vi "PicoScope2000ExampleAWG.vi"() -> ()   [LabVIEW 2010]
panel:
  in  "Waveform Settings":T1={"Arbirary waveform file path"=path "", "Sweep Type"=0, "Sweeps"=0, "Wave Type"=0, "Start Frequency"=1000.0, "Stop Frequency"=1000.0, "Increment (Hz)"=0.0, "Dwell Time (seconds)"=0.0, "Offset Voltage (uV)"=0, "Peak to Peak (uV)"=2000000} {"Start Frequency" min=1 max=1000000; "Wave Type" items=["Sine", "Square", "Triangle", "Ramp Up", "Ramp Down", "DC", "Arbitrary"]; "Sweep Type" items=["Up", "Down", "Up-Down", "Down-Up"]}
  in  "Apply Settings":bool
  in  "Stop VI":bool
  out "Arbitrary\nWaveform Graph":u8[](graph)
  # "Arbitrary waveform files must consist of a maximum\n4096 values, and should be in the range -1.0 (min. value) \nto +1.0 (max. value)."
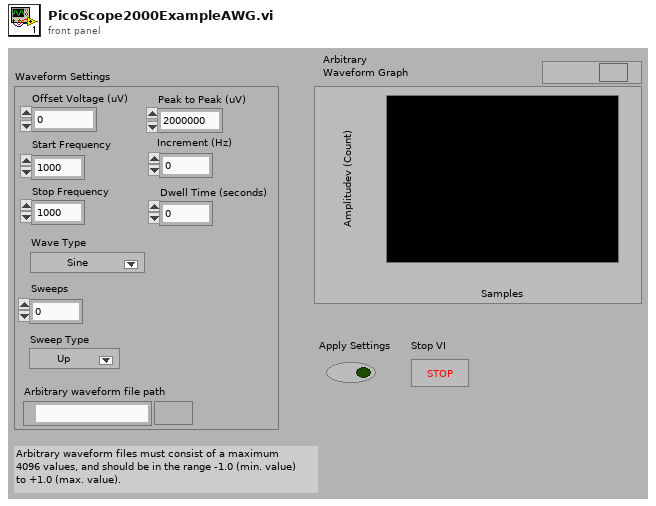
[diagram p1: front panel]
types:
  T1 = cluster{"Arbirary waveform file path":path, "Sweep Type":u32, "Sweeps":u32, "Wave Type":u32, "Start Frequency":sgl, "Stop Frequency":sgl, "Increment (Hz)":sgl, "Dwell Time (seconds)":sgl, "Offset Voltage (uV)":i32, "Peak to Peak (uV)":u32}
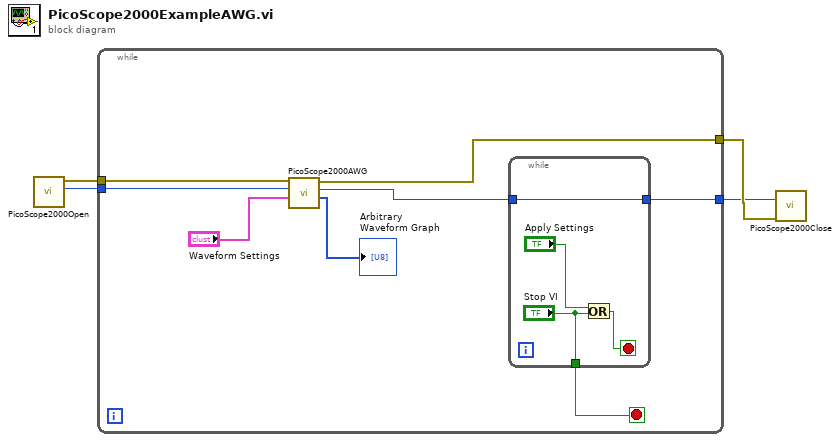
[diagram p0: block diagram]
diagram:
  n1 = call "PicoScope2000Open.vi"() -> ("handle"=w4:i16, "error out"=w3:errorcluster)  [unwired: 7 in, 1 out]
  n2 = while {
    tunnel: w4 -> [w11]
    tunnel: w3 -> [w10]
    tunnel: [w9] -> w1
    tunnel: [w7] -> w2
    stop <- w8 stop-if-true
    n3 = call "PicoScope2000AWG.vi"("Waveform Settings"="Waveform Settings", "Handle In"=w11, "error in"=w10) -> ("Arbitrary\nWaveform Graph"=→"Arbitrary\nWaveform Graph":u8[], "Handle Out"=w6:i16, "error out"=w7:errorcluster)  [unwired: 6 in]
    n4 = while {
      tunnel: ["Stop VI"] -> w8
      tunnel: [w16] -> w9
      tunnel: w6 -> [w16]
      stop <- w15 stop-if-true
      n5 = Or(x="Apply Settings", y="Stop VI") -> (x .or. y?=w15:bool)
    }
  }
  n6 = call "PicoScope2000Close.vi"("error in"=w2, "handle"=w1) -> ()  [unwired: 4 in, 2 out]
